vi "Picolog Get Last Error.vi"(8 "Error In":errorcluster, 11 "Instrument Handle In":i16=1) -> (0 "Error Out":errorcluster, 1 "Error Code":i16, 3 "Instrument Handle Out":i16)   [LabVIEW 2017]
uses:
  usbtc08.dll
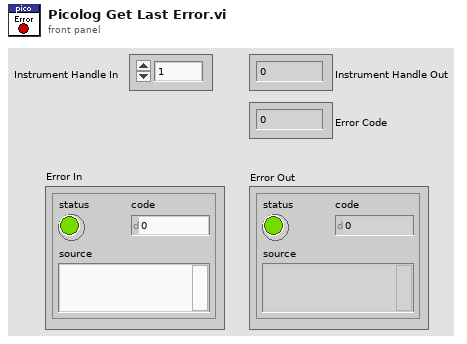
[diagram p1: front panel]
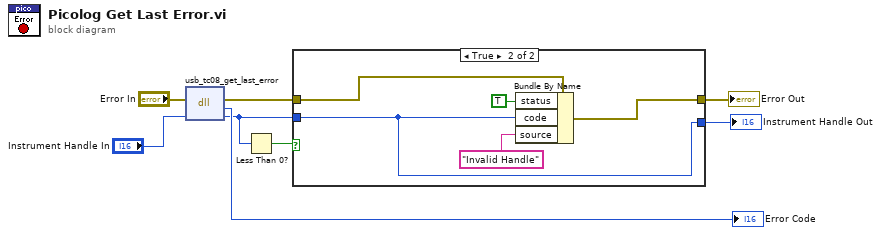
[diagram p0: block diagram]
diagram:
  n1 = dll-call lib="usbtc08.dll" fn="usb_tc08_get_last_error" label="OpenUnit"(error in="Error In", "handle"="Instrument Handle In") -> (error out=w8:errorcluster, "error_code"=→"Error Code":i16, "handle"=w1:i16)  [unwired: 2 in, 1 out]
  n2 = Less Than 0?(x=w1) -> (x < 0?=w5:bool)
  n3 = case shown="True" w5 {
    tunnel: w8 -> [w9 w14]
    tunnel: [w9 w15] -> w7
    tunnel: w1 -> [w10 w11]
    tunnel: [w10 w11] -> w3
    frame False {
    }
    frame True {
      n4 = Bundle By Name(cluster=w14, "status"=TRUE, "code"=w11, "source"="Invalid Handle") -> (w15:errorcluster)
    }
  }
  "Error Out" <- w7
  "Instrument Handle Out" <- w3
